vi "Load Config.vi"(8 "error in (no error)":errorcluster) -> (0 "error out":errorcluster, 3 "Array":T3(array[cluster]))   [LabVIEW 2020, in "Modbus.lvlib" / "Modbus.lvclass"]
uses:
  Modbus.lvclass
  Modbus Control Shortcut.ctl
  Modbus Channel Type.ctl
  Modbus Command Message.ctl
  <vilib>/Utility/config.llb/Read Key (String).vi
  <vilib>/Utility/config.llb/Read Key (I32).vi
  <vilib>/Utility/config.llb/NI_LVConfig.lvlib
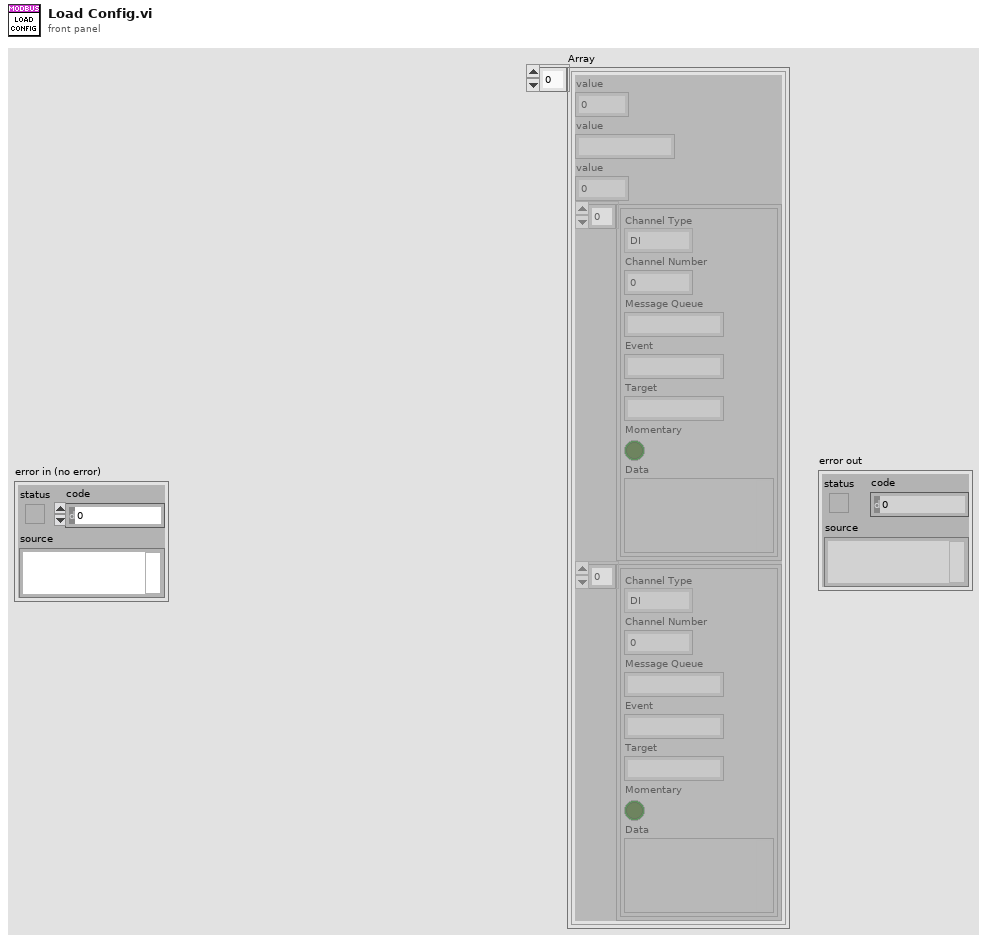
[diagram p1: front panel]
types:
  T1 = typedef "Modbus.lvlib/Modbus.lvclass/Modbus Control Shortcut.ctl" = cluster{"Channel Type":T2, "Channel Number":u8, "Message Queue":string, "Event":string, "Target":string, "Momentary":bool, "Data":variant}
  T2 = typedef "Modbus.lvlib/Modbus.lvclass/Modbus Channel Type.ctl" = enum16{"DI", "AI"}
  T3 = cluster{"value":i32, "value":string, "value":i32, T1[], T1[]}[]
  T4 = typedef "NI_LVConfig.lvlib/Config Data RefNum.ctl" = refnum<k1>
  T5 = typedef "Modbus.lvlib/Modbus.lvclass/Modbus Command Message.ctl" = cluster{"Command":string, "Message Queue":string, "Event":string, "Target":string, "Momentary":bool, "Data":variant}
  T6 = cluster{"value":i32, "value":string, "value":i32, T1[], T1[]}
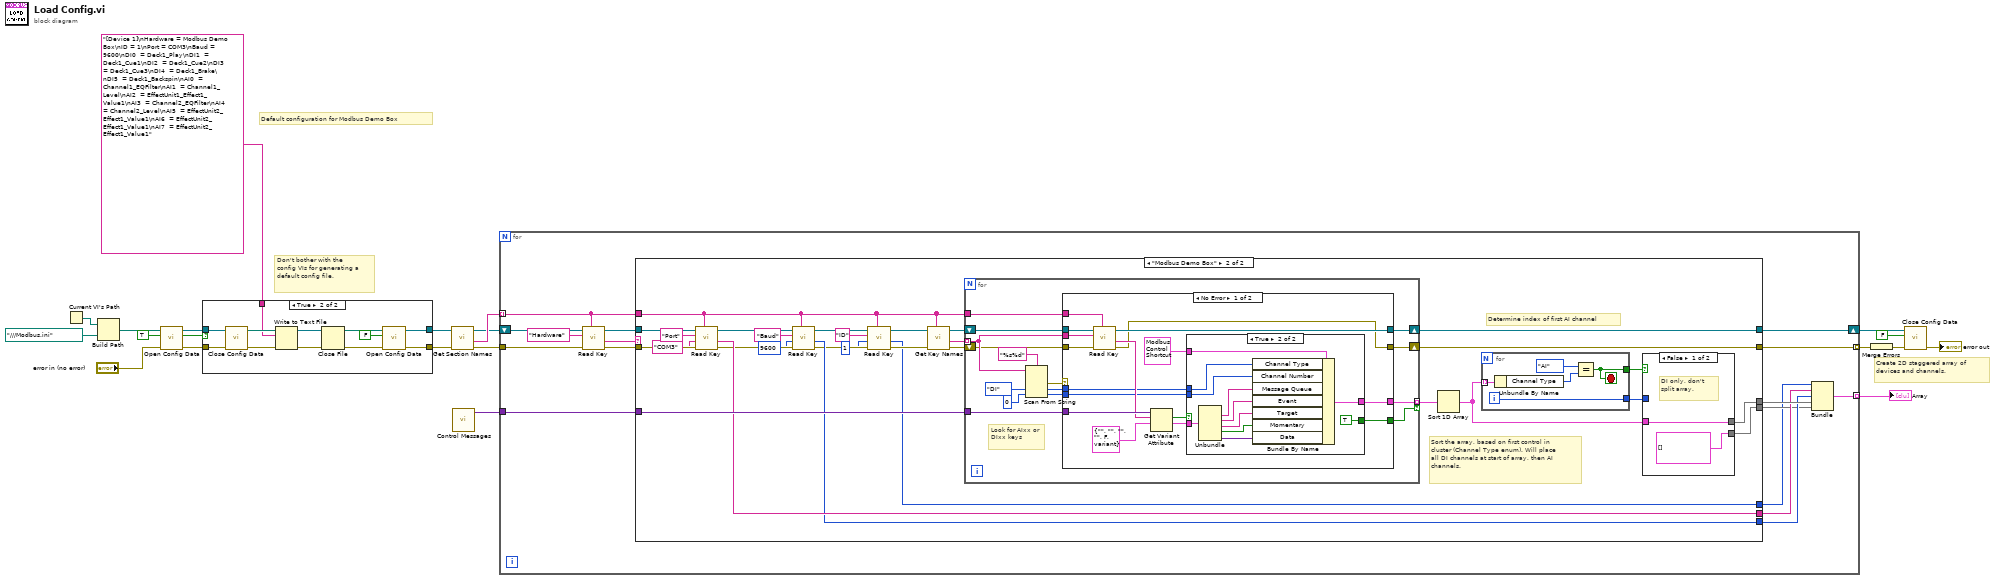
[diagram p0: block diagram]
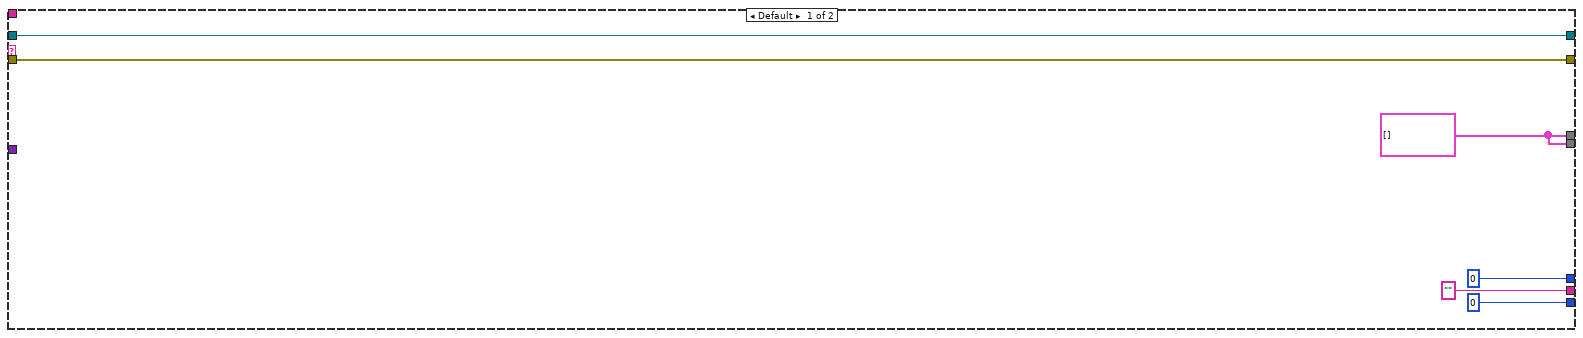
[diagram p3: hidden frame]
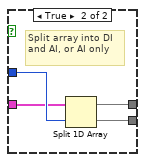
[diagram p4: hidden frame]
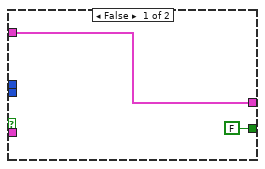
[diagram p5: hidden frame]
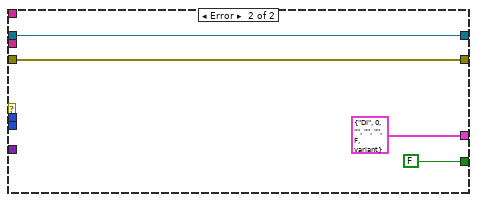
[diagram p6: hidden frame]
diagram:
  # "Don't bother with the config VIs for generating a default config file."
  # "Create 2D staggered array of devices and channels."
  # "Default configuration for Modbus Demo Box"
  n1 = Current VI's Path() -> (path=w13:path)
  n2 = Build Path(base path=w13, name or relative path=path "../../../Modbus.ini" ("configuration file path")) -> (appended path=w11:path)
  n3 = call <vilib>:"Open Config Data.vi"("error in (no error)"="error in (no error)", "create file if necessary (T)"=TRUE, "configuration file path"=w11) -> ("error out"=w6:errorcluster, "file created?"=w10:bool, "refnum"=w9:T4)  [unwired: 6 in]
  n4 = case shown="True" w10 {
    tunnel: w9 -> [w23 w35]
    tunnel: [w23 w24] -> w8
    tunnel: [w22 w25] -> w7
    tunnel: w6 -> [w22 w34]
    tunnel: "[Device 1]\nHardware = Modbus Demo Box\nID = 1\nPort = COM3\nBaud = 9600\nDI0  = Deck1_Play\nDI1  = Deck1_Cue1\nDI2  = Deck1_Cue2\nDI3  = Deck1_Cue3\nDI4  = Deck1_Brake\nDI5  = Deck1_Backspin\nAI0  = Channel1_EQFilter\nAI1  = Channel1_Level\nAI2  = EffectUnit1_Effect1_Value1\nAI3  = Channel2_EQFilter\nAI4  = Channel2_Level\nAI5  = EffectUnit2_Effect1_Value1\nAI6  = EffectUnit2_Effect1_Value1\nAI7  = EffectUnit2_Effect1_Value1" -> [_ w32]
    frame False {
    }
    frame True {
      n5 = call <vilib>:"Close Config Data.vi"("error in (no error)"=w34, "refnum"=w35) -> ("error out"=w31:errorcluster, "file path"=w33:path)  [unwired: 8 in]
      n6 = Write to Text File(file (use dialog)=w33, text=w32, error in=w31) -> (refnum out=w30:refnum<file>, error out=w29:errorcluster)  [unwired: 1 in, 1 out]
      n7 = Close File(refnum=w30, error in=w29) -> (path=w28:path, error out=w26:errorcluster)
      n8 = call <vilib>:"Open Config Data.vi"("error in (no error)"=w26, "create file if necessary (T)"=FALSE, "configuration file path"=w28) -> ("error out"=w25:errorcluster, "refnum"=w24:T4)  [unwired: 6 in, 1 out]
    }
  }
  n9 = call <vilib>:"Get Section Names.vi"("error in (no error)"=w7, "refnum"=w8) -> ("error out"=w17:errorcluster, "section names"=w19:string[], "refnum out"=w18:T4)  [unwired: 7 in]
  n10 = call "Control Messages.vi"() -> ("Shortcuts"=w20:variant)  [unwired: 11 in]
  n11 = for {
    tunnel: w19 -> [w47] mode=indexing
    tunnel: w17 -> [w39]
    shift-right: [w45] -> w15
    shift-left: w18 -> [w51]
    tunnel: w20 -> [w46]
    tunnel: [w43] -> w16 mode=indexing
    tunnel: [w37] -> w2 mode=indexing
    n12 = call-poly <vilib>:"Read Key.vi"("section"=w47, "error in (no error)"=w39, "key"="Hardware", "refnum"=w51) -> ("error out"=w38:errorcluster, "value"=w49:string, "refnum out"=w48:T4)  [unwired: 4 in, 1 out]
    n13 = case shown="\"Modbus Demo Box\"" w49 {
      tunnel: w48 -> [w57 w87]
      tunnel: w47 -> [_ w66]
      tunnel: w46 -> [_ w81]
      tunnel: [w57 w79] -> w45
      tunnel: [w56 w73] -> w44
      tunnel: ["" ("value") w78] -> w42
      tunnel: [0 ("value") w77] -> w41
      tunnel: [w56 w72] -> w40
      tunnel: w38 -> [w53 w71]
      tunnel: [w53 w68] -> w37
      tunnel: [0 ("value") w58] -> w36
      frame Default {
        w56 = T1[] []
      }
      frame "Modbus Demo Box" {
        # "Determine index of first AI channel"
        # "Sort the array, based on first control in cluster (Channel Type enum). Will place all DI channels at start of array, then AI channels."
        n14 = call-poly <vilib>:"Read Key.vi"("section"=w66, "error in (no error)"=w71, "default value"="COM3", "key"="Port", "refnum"=w87) -> ("error out"=w69:errorcluster, "value"=w78:string, "refnum out"=w85:T4)  [unwired: 3 in, 1 out]
        n15 = call-poly <vilib>:"Read Key.vi"("section"=w66, "error in (no error)"=w69, "default value"=9600, "key"="Baud", "refnum"=w85) -> ("error out"=w65:errorcluster, "value"=w77:i32, "refnum out"=w63:T4)  [unwired: 3 in, 1 out]
        n16 = call-poly <vilib>:"Read Key.vi"("section"=w66, "error in (no error)"=w65, "default value"=1, "key"="ID", "refnum"=w63) -> ("error out"=w64:errorcluster, "value"=w58:i32, "refnum out"=w62:T4)  [unwired: 3 in, 1 out]
        n17 = call <vilib>:"Get Key Names.vi"("section"=w66, "error in (no error)"=w64, "refnum"=w62) -> ("error out"=w67:errorcluster, "key names"=w83:string[], "refnum out"=w82:T4)  [unwired: 5 in, 1 out]
        n18 = for {
          tunnel: w83 -> [w110] mode=indexing
          shift-right: [w111] -> w79
          shift-left: w82 -> [w112]
          tunnel: w66 -> [w105]
          tunnel: w81 -> [w104]
          tunnel: [w102] -> w80 mode=indexing if=w101
          shift-right: [w100] -> w68
          shift-left: w67 -> [w99]
          # "Look for AIxx or DIxx keys"
          n19 = Scan From String(format string="%s%d", input string=w110, default 1=Modbus_Channel_Type."DI" ("Channel Type"), default 2=u8 0 ("default value 2")) -> (error out=w108:errorcluster, output 1=w107:T2, output 2=w106:u8)  [unwired: 2 in, 2 out]
          n20 = case shown="No Error" w108 {
            tunnel: w112 -> [w129 w145]
            tunnel: [w128 w145] -> w111
            tunnel: w110 -> [w127 _]
            tunnel: w107 -> [w120 _]
            tunnel: w106 -> [w119 _]
            tunnel: w105 -> [w126 _]
            tunnel: w104 -> [w125 _]
            tunnel: [w118 T1 {"Channel Type"=enum."DI", "Channel Number"=0, "Message Queue"="", "Event"="", "Target"="", "Momentary"=FALSE, "Data"=variant} ("DAQmx Shortcut")] -> w102
            tunnel: [w117 FALSE] -> w101
            tunnel: w99 -> [w115 w143]
            tunnel: [w114 w143] -> w100
            frame No Error {
              n21 = call-poly <vilib>:"Read Key.vi"("section"=w126, "error in (no error)"=w115, "key"=w127, "refnum"=w129) -> ("error out"=w114:errorcluster, "value"=w124:string, "refnum out"=w128:T4)  [unwired: 4 in, 1 out]
              n22 = Get Variant Attribute(Variant=w125, name=w124, default value (empty Variant)=T5 {"Command"="", "Message Queue"="", "Event"="", "Target"="", "Momentary"=FALSE, "Data"=variant} ("LINX Command Message")) -> (found=w116:bool, value=w121:T5)  [unwired: 1 in, 2 out]
              n23 = case shown="True" w116 {
                tunnel: T1 {"Channel Type"=enum."AI", "Channel Number"=0, "Message Queue"="Mixer", "Event"="Value Change", "Target"="Crossfader", "Momentary"=FALSE, "Data"=variant} ("LINX Control Shortcut") -> [w131 w142]
                tunnel: w121 -> [_ w141]
                tunnel: w120 -> [_ w140]
                tunnel: w119 -> [_ w139]
                tunnel: [w131 w133] -> w118
                tunnel: [FALSE TRUE] -> w117
                frame False {
                }
                frame True {
                  n24 = Unbundle(w141) -> ("Message Queue"=w138:string, "Event"=w137:string, "Target"=w136:string, "Momentary"=w135:bool, "Data"=w134:variant)  [unwired: 1 out]
                  n25 = Bundle By Name(cluster=w142, "Channel Type"=w140, "Channel Number"=w139, "Message Queue"=w138, "Event"=w137, "Target"=w136, "Momentary"=w135, "Data"=w134) -> (w133:T1)
                }
              }
            }
            frame Error {
            }
          }
        }
        n26 = Sort 1D Array(array=w80) -> (sorted array=w74:T1[])
        n27 = for {
          tunnel: w74 -> [w95] mode=indexing
          tunnel: [w97] -> w75
          tunnel: [w96] -> w76
          i -> [w97]
          stop <- w96 stop-if-true
          n28 = Unbundle By Name(w95) -> ("Channel Type"=w94:T2)
          n29 = Equal?(x=Modbus_Channel_Type."AI", y=w94) -> (x = y?=w96:bool)
        }
        n30 = case shown="False" w76 {
          tunnel: w75 -> [_ w93]
          tunnel: w74 -> [w89 w92]
          tunnel: [w89 w91] -> w73
          tunnel: [T1[] [] w90] -> w72
          frame False {
            # "DI only, don't split array."
          }
          frame True {
            # "Split array into DI and AI, or AI only"
            n31 = Split 1D Array(array=w92, index=w93) -> (first subarray=w91:T1[], second subarray=w90:T1[])
          }
        }
      }
    }
    n32 = Bundle("value"=w36, "value"=w42, "value"=w41, w44, w40) -> (w43:T6)  [unwired: 1 in]
  }
  "Array" <- w16
  n33 = Merge Errors(w2) -> (w1:errorcluster)
  n34 = call <vilib>:"Close Config Data.vi"("error in (no error)"=w1, "write file if changed (T)"=FALSE, "refnum"=w15) -> ("error out"=→"error out":errorcluster)  [unwired: 7 in, 1 out]
